vi "CH1_Comm_ZEROMQ.vi"() -> ()   [LabVIEW 2018]
uses:
  RxTx/RxTx.lvclass
  <vilib>/addons/zeromq/socket_type.ctl
  <vilib>/addons/zeromq/zmq_context.lvclass
  <vilib>/addons/zeromq/zeromq.lvlib
  <vilib>/addons/zeromq/zmq_socket.lvclass
panel:
  out "error out 4":errorcluster
  out "error out":errorcluster
  in  "stop":bool
  out "error out 3":errorcluster
  out "error out 2":errorcluster
  in  "RxTx.lvclass 2":refnum<class "RxTx.lvclass">
  in  "Channel":u16=1
  # "Channel 1 - TCPIP Communication"
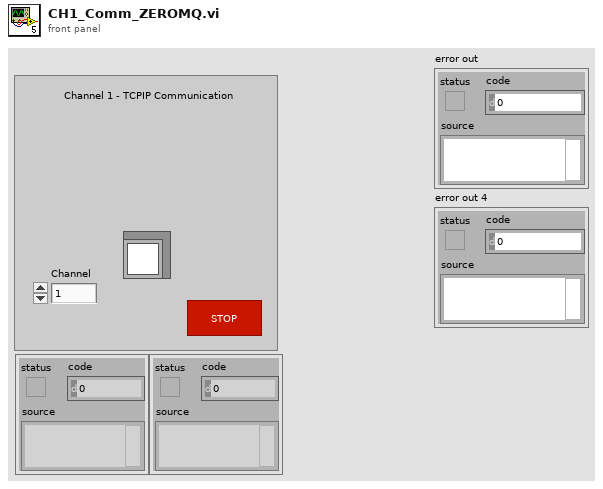
[diagram p1: front panel]
types:
  T1 = typedef "zeromq.lvlib/socket_type.ctl" = enum8{"ZMQ_PAIR", "ZMQ_PUB", "ZMQ_SUB", "ZMQ_REQ", "ZMQ_REP", "ZMQ_DEALER", "ZMQ_ROUTER", "ZMQ_PULL", "ZMQ_PUSH", "ZMQ_XPUB", "ZMQ_XSUB", "ZMQ_STREAM", "ZMQ_SERVER", "ZMQ_CLIENT", "ZMQ_RADIO", "ZMQ_DISH", "ZMQ_GATHER", "ZMQ_SCATTER", "ZMQ_DGRAM"}
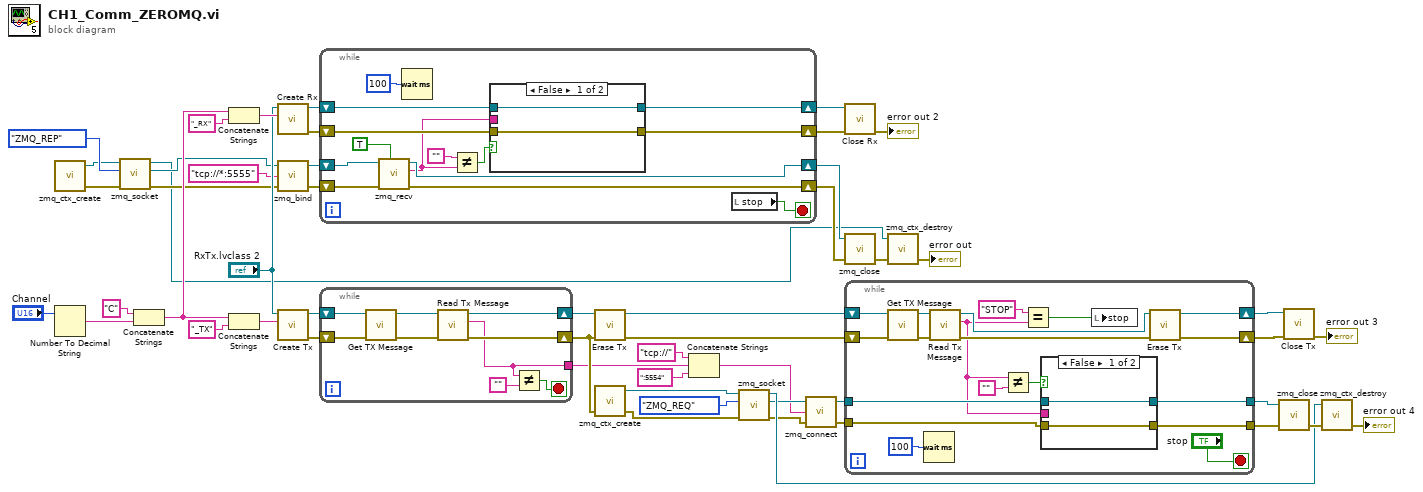
[diagram p0: block diagram]
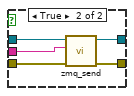
[diagram p2: hidden frame]
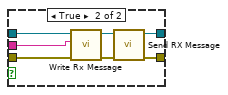
[diagram p3: hidden frame]
diagram:
  n1 = call <vilib>:"zmq_ctx_create.vi"() -> ("error out"=w31:errorcluster, "context out"=w32:refnum<class "zmq_context.lvclass">)  [unwired: 4 in]
  n2 = Number To Decimal String(number="Channel") -> (decimal integer string=w30:string)  [unwired: 1 in]
  n3 = call <vilib>:"zmq_socket.vi"("error in"=w31, "socket type"=socket_type."ZMQ_REP", "context in"=w32) -> ("error out"=w34:errorcluster, "socket out"=w35:refnum<class "zmq_socket.lvclass">, "context out"=w24:refnum<class "zmq_context.lvclass">)  [unwired: 2 in]
  n4 = Concatenate Strings("C", w30) -> (w38:string)
  n5 = Concatenate Strings(w38, "_RX" ("Reader Name")) -> (w52:string)
  n6 = Concatenate Strings(w38, "_TX" ("Reader Name")) -> (w44:string)
  n7 = call "Create Rx.vi"("Reader Name"=w52, "RxTx in"="RxTx.lvclass 2") -> ("error out"=w48:errorcluster, "RxTx out"=w49:refnum<class "RxTx.lvclass">)  [unwired: 8 in]
  n8 = call <vilib>:"zmq_bind.vi"("error in"=w34, "endpoint"="tcp://*:5555", "socket in"=w35) -> ("error out"=w29:errorcluster, "socket out"=w28:refnum<class "zmq_socket.lvclass">)  [unwired: 1 in]
  n9 = call "Create Tx.vi"("Writer Name"=w44, "RxTx in"="RxTx.lvclass 2") -> ("error out"=w10:errorcluster, "RxTx out"=w11:refnum<class "RxTx.lvclass">)  [unwired: 8 in]
  n10 = while {
    shift-right: [w61] -> w46
    shift-left: w48 -> [w66]
    shift-right: [w62] -> w47
    shift-left: w49 -> [w65]
    shift-right: [w57] -> w26
    shift-left: w28 -> [w58]
    shift-right: [w56] -> w25
    shift-left: w29 -> [w59]
    stop <- w60 stop-if-true
    n11 = call <vilib>:"zmq_recv.vi"("no block? (F)"=TRUE, "error in"=w59, "socket in"=w58) -> ("error out"=w56:errorcluster, "data"=w55:string, "socket out"=w57:refnum<class "zmq_socket.lvclass">)  [unwired: 2 in, 2 out]
    n12 = Wait (ms)(milliseconds to wait=u32 100) -> ()  [unwired: 1 out]
    n13 = Not Equal?(x="", y=w55) -> (x != y?=w63:bool)
    n14 = case shown="False" w63 {
      tunnel: w66 -> [w67 w73]
      tunnel: w65 -> [w68 w72]
      tunnel: [w68 w71] -> w62
      tunnel: [w67 w70] -> w61
      tunnel: w55 -> [_ w69]
      frame False {
      }
      frame True {
        n15 = call "Write Rx Message.vi"("error in (no error)"=w73, "Rx Message"=w69, "RxTx in"=w72) -> ("error out"=w74:errorcluster, "RxTx out"=w75:refnum<class "RxTx.lvclass">)  [unwired: 7 in]
        n16 = call "Send RX Message.vi"("error in (no error)"=w74, "RxTx in"=w75) -> ("error out"=w70:errorcluster, "RxTx out"=w71:refnum<class "RxTx.lvclass">)  [unwired: 8 in]
      }
    }
    n17 = local read "stop"() -> (w60:bool)
  }
  n18 = while {
    shift-right: [w82] -> w9
    shift-left: w11 -> [w84]
    shift-right: [w81] -> w8
    shift-left: w10 -> [w79]
    tunnel: [w76] -> w6
    stop <- w77 stop-if-true
    n19 = call "Get TX Message.vi"("error in (no error)"=w79, "RxTx in"=w84) -> ("error out"=w80:errorcluster, "RxTx out"=w83:refnum<class "RxTx.lvclass">)  [unwired: 8 in]
    n20 = call "Read Tx Message.vi"("error in (no error)"=w80, "RxTx in"=w83) -> ("error out"=w81:errorcluster, "Tx Message"=w76:string, "RxTx out"=w82:refnum<class "RxTx.lvclass">)  [unwired: 7 in]
    n21 = Not Equal?(x=w76, y="") -> (x != y?=w77:bool)
  }
  n22 = call "Erase Tx.vi"("error in (no error)"=w8, "RxTx in"=w9) -> ("error out"=w36:errorcluster, "RxTx out"=w37:refnum<class "RxTx.lvclass">)  [unwired: 8 in]
  n23 = call <vilib>:"zmq_ctx_create.vi"("error in"=w8) -> ("error out"=w20:errorcluster, "context out"=w21:refnum<class "zmq_context.lvclass">)  [unwired: 3 in]
  n24 = Concatenate Strings("tcp://" ("endpoint"), w6, ":5554" ("endpoint")) -> (w1:string)
  n25 = call <vilib>:"zmq_socket.vi"("error in"=w20, "socket type"=socket_type."ZMQ_REQ", "context in"=w21) -> ("error out"=w3:errorcluster, "socket out"=w2:refnum<class "zmq_socket.lvclass">, "context out"=w16:refnum<class "zmq_context.lvclass">)  [unwired: 2 in]
  n26 = call <vilib>:"zmq_connect.vi"("error in"=w3, "endpoint"=w1, "socket in"=w2) -> ("error out"=w5:errorcluster, "socket out"=w4:refnum<class "zmq_socket.lvclass">)  [unwired: 1 in]
  n27 = call "Close Rx.vi"("error in (no error)"=w46, "RxTx in"=w47) -> ("error out"=→"error out 2":errorcluster)  [unwired: 8 in, 1 out]
  n28 = call <vilib>:"zmq_close.vi"("error in"=w25, "socket"=w26) -> ("error out"=w27:errorcluster)  [unwired: 3 in]
  n29 = while {
    shift-right: [w103] -> w42
    shift-left: w37 -> [w96]
    shift-right: [w102] -> w41
    shift-left: w36 -> [w95]
    tunnel: w4 -> [w91]
    tunnel: w5 -> [w90]
    tunnel: [w89] -> w18
    tunnel: [w88] -> w17
    stop <- "stop" stop-if-true
    n30 = call "Get TX Message.vi"("error in (no error)"=w95, "RxTx in"=w96) -> ("error out"=w101:errorcluster, "RxTx out"=w97:refnum<class "RxTx.lvclass">)  [unwired: 8 in]
    n31 = Wait (ms)(milliseconds to wait=u32 100) -> ()  [unwired: 1 out]
    n32 = call "Read Tx Message.vi"("error in (no error)"=w101, "RxTx in"=w97) -> ("error out"=w98:errorcluster, "Tx Message"=w87:string, "RxTx out"=w99:refnum<class "RxTx.lvclass">)  [unwired: 7 in]
    n33 = Not Equal?(x=w87, y="") -> (x != y?=w94:bool)
    n34 = Equal?(x="STOP" ("Reader Name"), y=w87) -> (x = y?=w85:bool)
    n35 = case shown="False" w94 {
      tunnel: w87 -> [_ w106]
      tunnel: w91 -> [w105 w110]
      tunnel: w90 -> [w104 w109]
      tunnel: [w105 w108] -> w89
      tunnel: [w104 w107] -> w88
      frame False {
      }
      frame True {
        n36 = call <vilib>:"zmq_send.vi"("error in"=w109, "data"=w106, "socket in"=w110) -> ("error out"=w107:errorcluster, "socket out"=w108:refnum<class "zmq_socket.lvclass">)  [unwired: 4 in]
      }
    }
    n37 = local write "stop"(w85) -> ()
    n38 = call "Erase Tx.vi"("error in (no error)"=w98, "RxTx in"=w99) -> ("error out"=w102:errorcluster, "RxTx out"=w103:refnum<class "RxTx.lvclass">)  [unwired: 8 in]
  }
  n39 = call <vilib>:"zmq_ctx_destroy.vi"("error in"=w27, "context in"=w24) -> ("error out"=→"error out":errorcluster)  [unwired: 3 in]
  n40 = call <vilib>:"zmq_close.vi"("error in"=w17, "socket"=w18) -> ("error out"=w19:errorcluster)  [unwired: 3 in]
  n41 = call "Close Tx.vi"("error in (no error)"=w41, "RxTx in"=w42) -> ("error out"=→"error out 3":errorcluster)  [unwired: 8 in, 1 out]
  n42 = call <vilib>:"zmq_ctx_destroy.vi"("error in"=w19, "context in"=w16) -> ("error out"=→"error out 4":errorcluster)  [unwired: 3 in]
